vi "Delete Multiple Symbol Notifications.vi"(7 "Aliases":string[](array[string]), 8 "error in (no error)":errorcluster, 10 "Symbol Names":string[](array[string]), 11 "TwinCAT ADS in":refnum<class "TwinCAT ADS.lvclass">) -> (0 "error out":errorcluster, 3 "TwinCAT ADS out":refnum<class "TwinCAT ADS.lvclass">)   [LabVIEW 2018, in "TwinCAT ADS.lvclass"]
uses:
  TwinCAT ADS.lvclass
  TwinCAT ADS.lvclass/TwinCAT ADS.ctl
  Delete Notification From Map.vi
  Get Notification Map.vi
  To Notification Key.vi
  <vilib>/Utility/error.llb/Trim Whitespace.vi
  Extensions/Delete Notification By Handle.vi
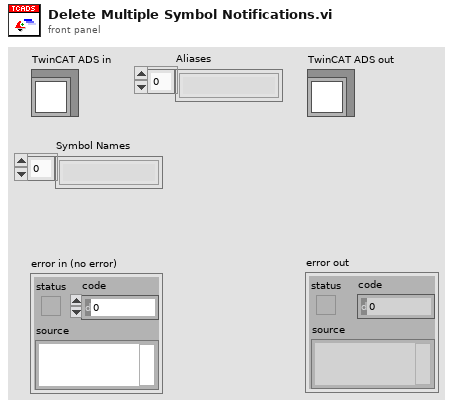
[diagram p1: front panel]
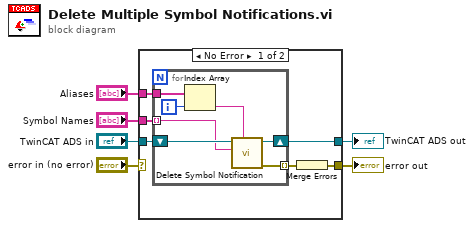
[diagram p0: block diagram]
diagram:
  n1 = case shown="No Error" "error in (no error)" {
    selector: "error in (no error)" -> [_ w21]
    tunnel: [w8 w21] -> w5
    tunnel: [w9 w20] -> w3
    tunnel: "TwinCAT ADS in" -> [w12 w20]
    tunnel: "Symbol Names" -> [w11 _]
    tunnel: "Aliases" -> [w7 _]
    frame No Error {
      n2 = for {
        shift-right: [w18] -> w9
        shift-left: w12 -> [w19]
        tunnel: [w17] -> w10 mode=indexing
        tunnel: w11 -> [w16] mode=indexing
        tunnel: w7 -> [w15]
        i -> [w14]
        n3 = Index Array(array=w15, index=w14) -> (element=w13:string)
        n4 = call "Delete Symbol Notification.vi"("Alias"=w13, "Symbol Name"=w16, "TwinCAT ADS in"=w19) -> ("error out"=w17:errorcluster, "TwinCAT ADS out"=w18:refnum<class "TwinCAT ADS.lvclass">)  [unwired: 7 in]
      }
      n5 = Merge Errors(w10) -> (w8:errorcluster)
    }
    frame Error {
    }
  }
  "error out" <- w5
  "TwinCAT ADS out" <- w3
